vi "Kalman filter - Angle & Bias(SubVI).vi"(2 "Bias in":dbl, 3 "Angle in":dbl, 4 "Accelerometer":dbl, 5 "K Array in":dbl[](array[numeric])) -> (0 "Bias out":dbl, 1 "Angle out":dbl)   [LabVIEW 2013]
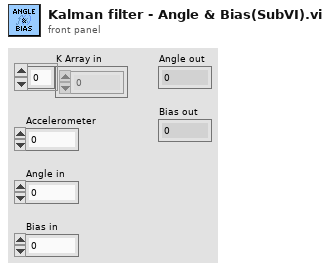
[diagram p1: front panel]
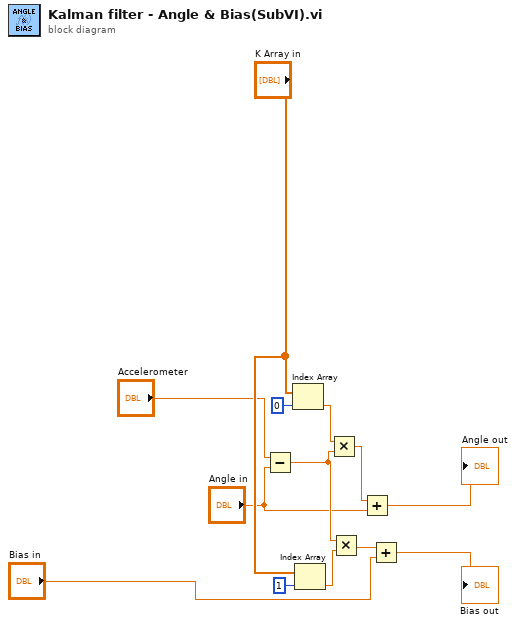
[diagram p0: block diagram]
diagram:
  n1 = Subtract(x="Accelerometer", y="Angle in") -> (x-y=w10:dbl)
  n2 = Index Array(array="K Array in", index=0) -> (element=w3:dbl)
  n3 = Index Array(array="K Array in", index=1) -> (element=w9:dbl)
  n4 = Multiply(x=w3, y=w10) -> (x*y=w4:dbl)
  n5 = Multiply(x=w10, y=w9) -> (x*y=w11:dbl)
  n6 = Add(x=w4, y="Angle in") -> (x+y=→"Angle out":dbl)
  n7 = Add(x=w11, y="Bias in") -> (x+y=→"Bias out":dbl)
